vi "Primary logic for trip prevention.vi"(8 "VISA Refnum in":refnum<visa-resource-name>) -> ()   [LabVIEW 2020]
uses:
  <instrlib>/CAEN PSM/CAEN PSM.lvlib
panel:
  out "BoardHandle out":T1
  out "error out":errorcluster
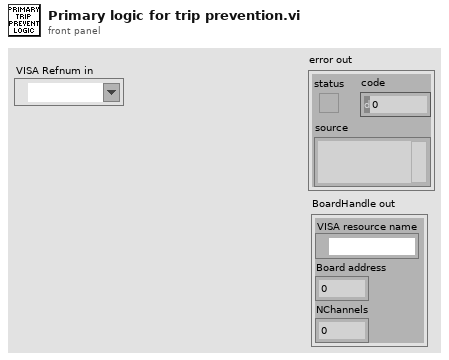
[diagram p1: front panel]
types:
  T1 = cluster{"VISA resource name":refnum<visa-resource-name>, "Board address":u8, "NChannels":u8}
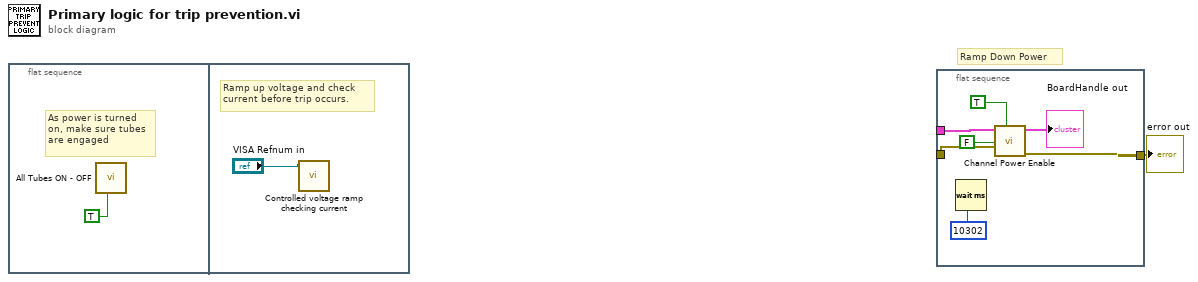
[diagram p0: block diagram]
diagram:
  # "Ramp Down Power"
  n1 = flat-sequence {
    frame #0 {
      # "As power is turned\non, make sure tubes\nare engaged"
      n2 = call "All Tubes ON - OFF.vi"("Tubes ON/OFF"=TRUE ("Activate: 1\nDeactivate: 0")) -> ()  [unwired: 11 in]
    }
    frame #1 {
      # "Ramp up voltage and check \ncurrent before trip occurs."
      n3 = call "Controlled voltage ramp checking current.vi"("VISA Refnum in"="VISA Refnum in") -> ()  [unwired: 9 in, 2 out]
    }
  }
  n4 = flat-sequence {
    tunnel: [w12] -> w1
    tunnel: [w11] -> w3
    tunnel: [w10] -> w2
    frame #0 {
      n5 = Wait (ms)(milliseconds to wait=u32 10302) -> ()  [unwired: 1 out]
      n6 = call <instrlib>:"Channel Power Enable.vi"("All Channels (F)"=TRUE, "error in (no error)"=w12, "Enable (OFF)"=FALSE, "BoardHandle"=w11) -> ("error out"=w10:errorcluster, "BoardHandle out"=→"BoardHandle out":T1)  [unwired: 6 in]
    }
  }
  "error out" <- w2
